vi "Pre-Build Action.vi"(6 "Top Level/Always Included VIs":path[](array[path]), 7 "Main Destination Path":path, 9 "Target Name":string, 10 "Build Specification Name":string, 11 "Project Path":path) -> (0 "error out":errorcluster)   [LabVIEW 2019, in "Launcher Support.lvlib"]
doc: "This Pre-Build Action VI sets the Debug mode to false to ensure the top level VI has the headless properties at build time.\n_____\nBased on DQMH Project Template 6.1.0.94."
uses:
  Launcher Support.lvlib
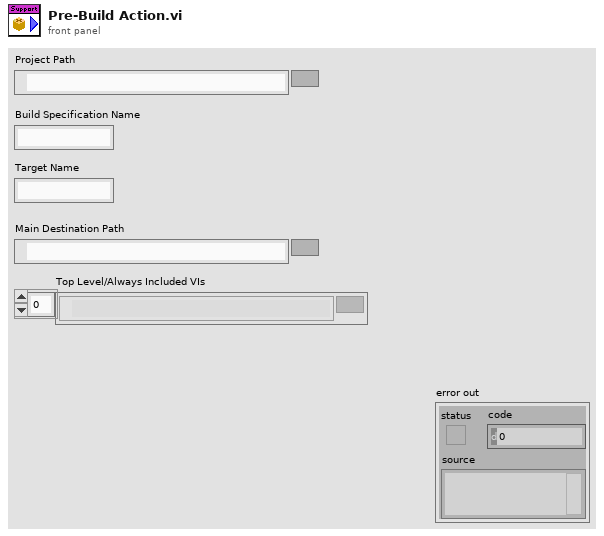
[diagram p1: front panel]
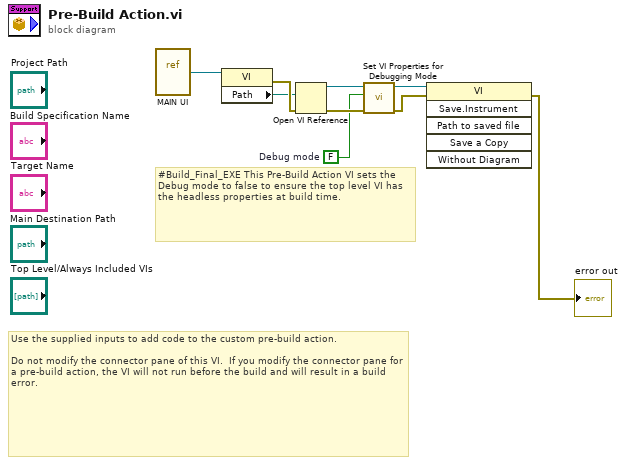
[diagram p0: block diagram]
diagram:
  w4 = FALSE  # Debug mode
  # "#Build_Final_EXE This Pre-Build Action VI sets the Debug mode to false to ensure the top level VI has the headless properties at build time."
  # "Use the supplied inputs to add code to the custom pre-build action.\n\nDo not modify the connector pane of this VI.  If you modify the connector pane for a pre-build action, the VI will not run before the build and will result in a build error."
  n1 = vi-ref "MAIN UI.vi"() -> (w7:refnum<vi>)
  n2 = property class="VI"(reference=w7) -> (error out=w9:errorcluster, "Path"=w6:path)  [unwired: 1 in, 1 out]
  n3 = Open VI Reference(vi path=w6, error in (no error)=w9) -> (vi reference=w5:refnum<vi>, error out=w8:errorcluster)  [unwired: 4 in]
  n4 = call "Set VI Properties for Debugging Mode.vi"("error in (no error)"=w8, "Debug mode?"=w4, "Launcher VI ref"=w5) -> ("error out"=w1:errorcluster, "Launcher VI ref out"=w3:refnum<vi>)  [unwired: 7 in]
  n5 = invoke class="VI" method="Save.Instrument"(reference=w3, error in=w1) -> (error out=→"error out":errorcluster)  [unwired: 4 in, 5 out]
